vi "APC_9049_ControlSettingsPolling.vi"() -> (0 "9049_ControlSettings":dbl[](array[numeric]))   [LabVIEW 2020]
doc: "This example demonstrates the procedure required to apply different NI-DAQmx Custom Scales to each virtual channel in a task. A DAQmx Task Property Node (Functions >> NI Measurements >> DAQmx - Data Acquisition >> DAQmx Advanced Task Options) is used to obtain the task's virtual channels. A DAQmx Channel Property Node (Functions >> NI Measurements >> DAQmx - Data Acquisition) is then used to set the custom scale for each virtual channel in the task.\n\nThe \"DAQmx Create Scale\" VI creates a custom scale for each channel in the channel list. *Note, make sure your Minimum and Maximum channel parameters are consistent with the range the scale will create."
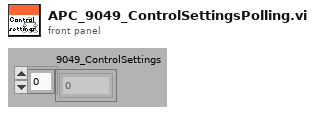
[diagram p1: front panel]
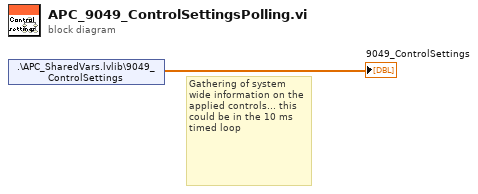
[diagram p0: block diagram]
diagram:
  # "Gathering of system wide information on the applied controls... this could be in the 10 ms timed loop"
  n1 = shared-variable ".\\APC_SharedVars.lvlib\\9049_ControlSettings"() -> (→"9049_ControlSettings":dbl[])  [unwired: 1 in, 1 out]
